vi "OpenReadWriteCloseSerial.vi"(10 "String":string, 11 "VISA Refnum in":refnum<visa-resource-name>(xcontrol)="ASRL1") -> (3 "reply":string)   [LabVIEW 2024]
uses:
  <userlib>/SerialVIs/subs/portX.xctl
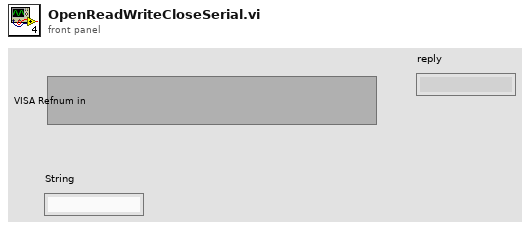
[diagram p1: front panel]
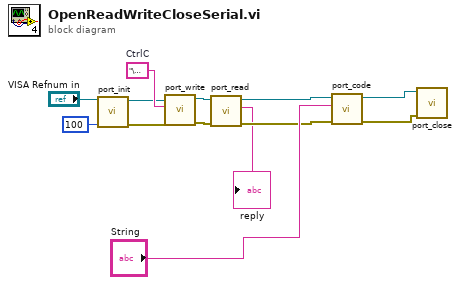
[diagram p0: block diagram]
diagram:
  w13 = "\u0003"  # CtrlC
  n1 = call <userlib>:"port_init.vi"("Timeout (ms)"=u32 100, "VISA Refnum in"="VISA Refnum in") -> ("error out"=w10:errorcluster, "VISA Refnum out"=w4:refnum<visa-resource-name>)  [unwired: 8 in]
  n2 = call <userlib>:"port_write.vi"("error in (no error)"=w10, "write buffer"=w13, "VISA Refnum in"=w4) -> ("error out"=w8:errorcluster, "VISA Refnum out"=w9:refnum<visa-resource-name>)  [unwired: 7 in]
  n3 = call <userlib>:"port_read.vi"("error in (no error)"=w8, "VISA Refnum in"=w9) -> ("error out"=w6:errorcluster, "reply"=→"reply":string, "VISA Refnum out"=w5:refnum<visa-resource-name>)  [unwired: 7 in]
  n4 = call <userlib>:"port_code.vi"("error in (no error)"=w6, "Code to run"="String", "VISA Refnum in"=w5) -> ("error out"=w2:errorcluster, "VISA Refnum out"=w3:refnum<visa-resource-name>)  [unwired: 7 in]
  n5 = call <userlib>:"port_close.vi"("error in (no error)"=w2, "VISA Refnum in"=w3) -> ()  [unwired: 10 in]
